vi "capture and save.vi"(11 "hwnd":u32) -> (3 "hwnd 2":u32)   [LabVIEW 2011]
uses:
  user32.dll
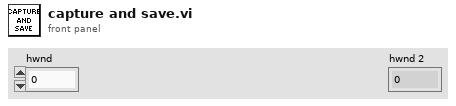
[diagram p1: front panel]
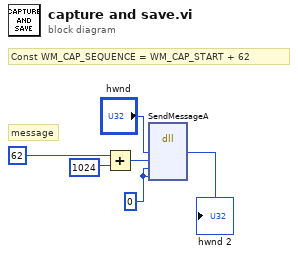
[diagram p0: block diagram]
diagram:
  w5 = u32 0 ("wParam")
  # "message"
  # "Const WM_CAP_SEQUENCE = WM_CAP_START + 62"
  n1 = Add(x=u32 62, y=u32 1024 ("msg")) -> (x+y=w3:u32)
  n2 = dll-call lib="user32.dll" fn="SendMessageA"("hwnd"="hwnd", "msg"=w3, "wParam"=w5, "lparam"=w5) -> ("hwnd"=→"hwnd 2":u32)  [unwired: 7 in, 2 out]
